vi "6進階題-ListBox.vi"() -> ()   [LabVIEW 2019]
panel:
  in  "Stop":bool
  out "Sum":i32
  in  "品名價格":i32[](listbox)=[4, 5]
  # "進階題：1. 以Multicolumn Listbox製作價目表如下，其中包含至少兩項無庫存；\n              2. 程式開始執行後，會自動將無庫存的項目Disable；\n              3. 使用者可複選不同的項目。選定項目的總價格會顯示在Sum中。"
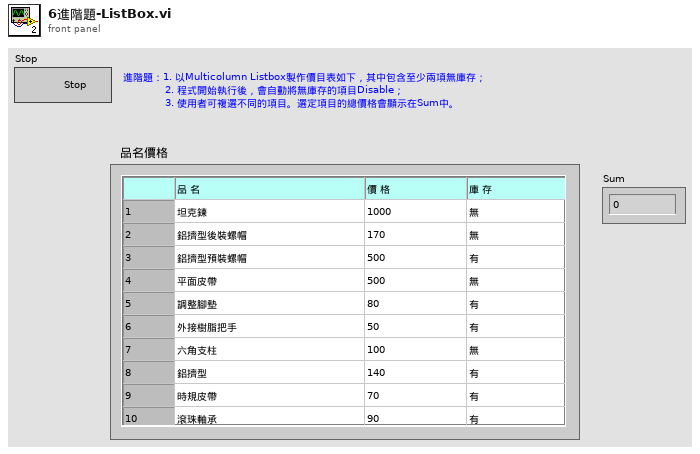
[diagram p1: front panel]
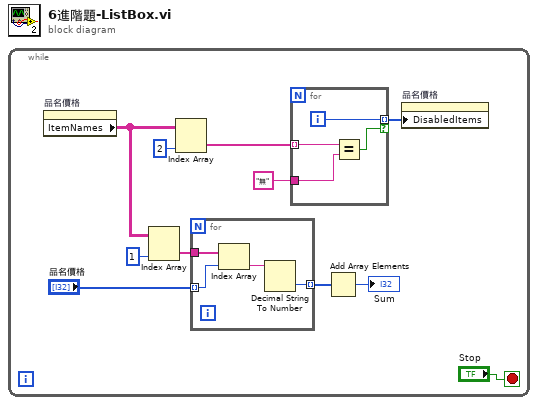
[diagram p0: block diagram]
diagram:
  n1 = while {
    stop <- "Stop" stop-if-true
    n2 = property on="品名價格" class="MCListbox (strict)"() -> ("ItemNames"=w6:string[][])  [unwired: 2 in, 2 out]
    n3 = Index Array(array=w6, index (col)=1 ("disabled index (col)")) -> (element=w5:string[])  [unwired: 1 in]
    n4 = Index Array(array=w6, index (col)=2 ("disabled index (col)")) -> (element=w11:string[])  [unwired: 1 in]
    n5 = for {
      tunnel: w5 -> [w15]
      tunnel: "品名價格" -> [w14] mode=indexing
      tunnel: [w12] -> w3 mode=indexing
      n6 = Index Array(array=w15, index=w14) -> (element=w13:string)
      n7 = Decimal String To Number(string=w13) -> (number=w12:i32)  [unwired: 2 in, 1 out]
    }
    n8 = for {
      tunnel: w11 -> [w19] mode=indexing
      tunnel: "無" ("y") -> [w18]
      tunnel: [w17] -> w8 mode=indexing if=w16
      i -> [w17]
      n9 = Equal?(x=w19, y=w18) -> (x = y?=w16:bool)
    }
    n10 = Add Array Elements(numeric array=w3) -> (sum=→"Sum":i32)
    n11 = property on="品名價格" class="MCListbox (strict)"("DisabledItems"=w8) -> ()  [unwired: 2 in, 2 out]
  }
